vi "ImagTest.vi"() -> ()   [LabVIEW 2014]
panel:
  in  "Color Palette":cluster{"Red":u8, "Green":u8, "Blue":u8}[](array[cluster])
  in  "TIFF Options":T1={"Rows Per Strip"=0, "Photometric"=1, "Compression Type"=0} {"Compression Type" items=["None", "JPEG", "Run Length Encoded", "Zip"]; "Photometric" items=["WhiteIsZero", "BlackIsZero"]}
  in  "X Resolution":i32
  in  "Y Resolution":i32
  out "error out":errorcluster
  out "Image":T2(plugin-control)
  out "Array":u16[][](array[numeric])
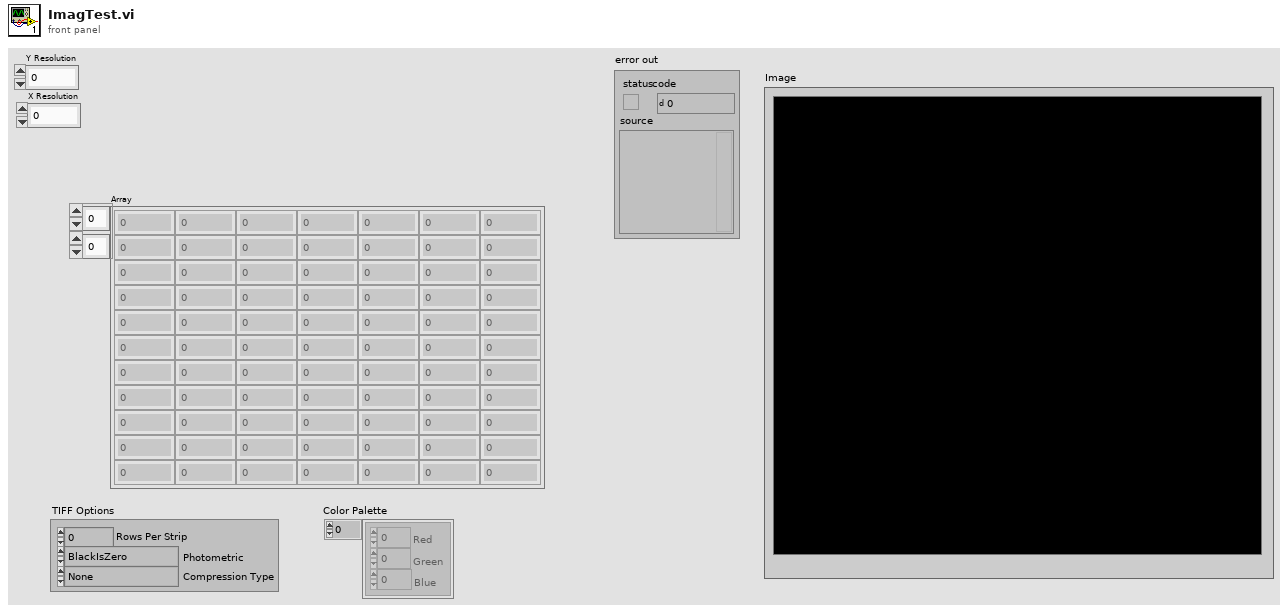
[diagram p1: front panel]
types:
  T1 = cluster{"Rows Per Strip":i32, "Photometric":i32, "Compression Type":i32}
  T2 = typedef "IMAQ Image.ctl" = refnum<image>
  T3 = typedef "Image Type" = u32
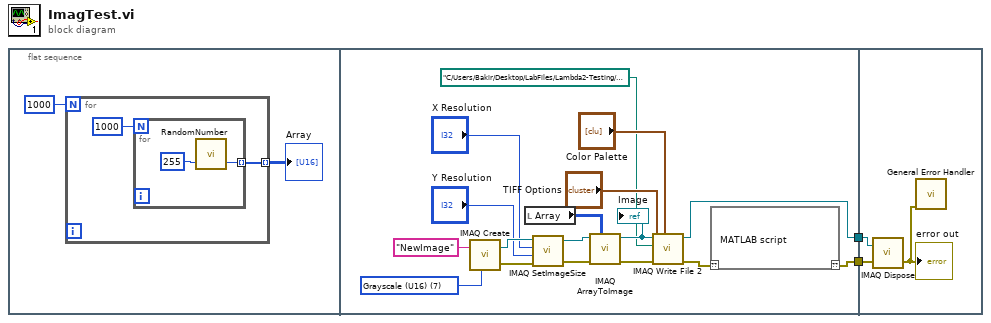
[diagram p0: block diagram]
diagram:
  n1 = flat-sequence {
    tunnel: [w11] -> w2
    tunnel: [w9] -> w1
    tunnel: w2 -> [w28]
    tunnel: w1 -> [w27]
    frame #0 {
      n2 = for {
        N: 1000 -> [_]
        tunnel: [w6] -> w4 mode=indexing
        n3 = for {
          N: 1000 -> [_]
          tunnel: [w7] -> w6 mode=indexing
          n4 = call <vilib>:"RandomNumber.vi"("Max Value"=255) -> ("Random Number"=w7:u16)  [unwired: 2 in, 1 out]
        }
      }
      "Array" <- w4
    }
    frame #1 {
      w24 = T3 7 items=["Grayscale (U8)", "Grayscale (I16)", "Grayscale (SGL)", "Complex (CSG)", "RGB (U32)", "HSL (U32)", "RGB (U64)", "Grayscale (U16)"] ("Image Type")
      n5 = call "IMAQ Create"("Image Name"="NewImage", "Image Type"=w24) -> ("New Image"=w17:T2, "error out"=w19:errorcluster)  [unwired: 3 in]
      n6 = local read "Array"() -> (w23:u16[][])
      n7 = call "IMAQ SetImageSize"("error in (no error)"=w19, "Y Resolution"="Y Resolution", "X Resolution"="X Resolution", "Image"=w17) -> ("error out"=w20:errorcluster, "Image Out"=w18:T2)  [unwired: 1 in]
      n8 = call "IMAQ ArrayToImage"("Image Pixels (U16)"=w23, "error in (no error)"=w20, "Image"=w18) -> ("error out"=w21:errorcluster, "Image Out"=w22:T2)  [unwired: 7 in]
      "Image" <- w22
      n9 = call-poly "IMAQ Write File 2"("Color Palette"="Color Palette", "error in (no error)"=w21, "TIFF Options"="TIFF Options", "File Path"=path "C:/Users/Bakir/Desktop/LabFiles/Lambda2-Testing/NewImage.tiff", "Image"=w22) -> ("error out"=w12:errorcluster, "Image Out (duplicate)"=w9:T2)  [unwired: 5 in]
      n10 = script code="MATLAB script"("??"=w12) -> ("??"=w11:errorcluster)
    }
    frame #2 {
      n11 = call "IMAQ Dispose"("Image"=w27, "error in (no error)"=w28) -> ("error out"=w26:errorcluster)  [unwired: 4 in]
      "error out" <- w26
      n12 = call <vilib>:"General Error Handler.vi"("error in (no error)"=w26) -> ()  [unwired: 10 in, 5 out]
    }
  }
